vi "Write to Cell - Dbl.vi"(8 "Column":i32=-1, 9 "Row":i32=-1, 10 "Value":dbl, 11 "Excel Sheet in":refnum<class "Excel Sheet.lvclass">) -> (3 "Excel Sheet out":refnum<class "Excel Sheet.lvclass">)   [LabVIEW 2016, in "Excel Sheet.lvclass"]
uses:
  Excel Sheet.lvclass
panel:
  out "error out":errorcluster
  in  "error in (no error)":errorcluster
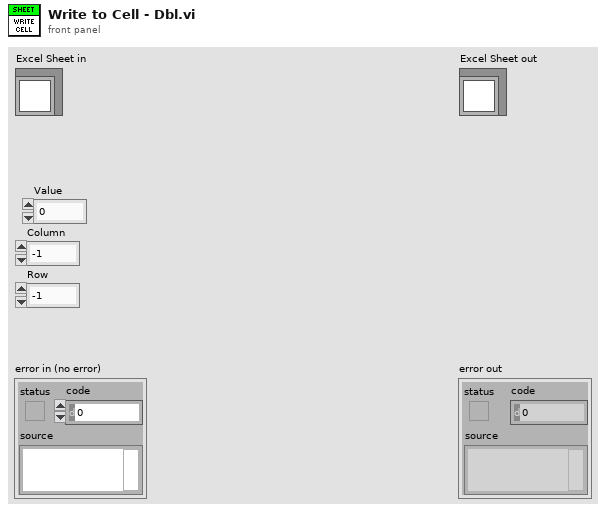
[diagram p1: front panel]
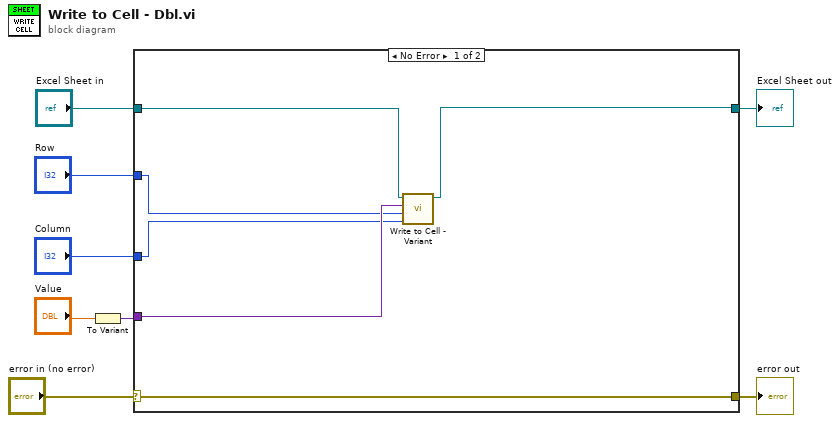
[diagram p0: block diagram]
diagram:
  n1 = To Variant(anything="Value") -> (Variant=w2:variant)
  n2 = case shown="No Error" "error in (no error)" {
    selector: "error in (no error)" -> [w14 w16]
    tunnel: [w14 w16] -> w7
    tunnel: [w12 w15] -> w5
    tunnel: "Excel Sheet in" -> [w13 w15]
    tunnel: "Column" -> [w9 _]
    tunnel: "Row" -> [w10 _]
    tunnel: w2 -> [w11 _]
    frame No Error {
      n3 = call "Write to Cell - Variant.vi"("Column"=w9, "Row"=w10, "Value"=w11, "Excel Sheet in"=w13) -> ("Excel Sheet out"=w12:refnum<class "Excel Sheet.lvclass">)  [unwired: 7 in]
    }
    frame Error {
    }
  }
  "error out" <- w7
  "Excel Sheet out" <- w5
